vi "onTestSlippage.vi"(7 "BananaPeel in":refnum<class "BananaPeel.lvclass">, 10 "Properties.Test":refnum<class "Properties.Test.lvclass">) -> (0 "error out":errorcluster, 2 "Properties.Test out":refnum<class "Properties.Test.lvclass">)   [LabVIEW 2021, in "Bananas.lvlib" / "BananaPeel.lvclass"]
uses:
  BananaPeel.lvclass
  <vilib>/addons/_JKI Toolkits/Caraya/classes/Properties.Test/Properties.Test.lvclass
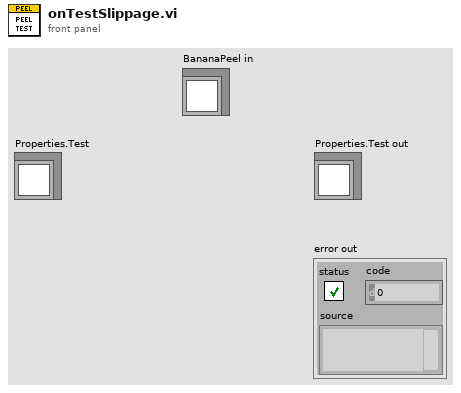
[diagram p1: front panel]
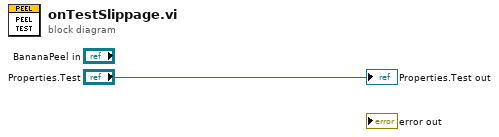
[diagram p0: block diagram]
diagram:
  "Properties.Test out" <- "Properties.Test"
